vi "Configure List Parameters.vi"(0 "VISA resource name":refnum<visa-resource-name>, 1 "List File Number (1)":dbl=1.0 min=1.0 max=10.0 step=1.0, 2 "Address (0)":dbl min=0.0 max=31.0 step=1.0 format="%#.0p", 5 "List Power Limit (1200)":dbl=1200.0 min=1.0 max=1200.0 step=1.0, 7 "Repeat Count (1)":i32=1 min=1 max=65535 step=1, 9 "Linked Sequences (0000000000)":bool[](array[boolean])=[FALSE, FALSE, FALSE, FALSE, FALSE, FALSE, FALSE, FALSE, FALSE, FALSE], 11 "error in (no error)":errorcluster) -> (4 "VISA resource name out":refnum<visa-resource-name>, 15 "error out":errorcluster)   [LabVIEW 2020, in "BK Precision 911X Series.lvlib"]
doc: "Configures list parameters for list operation. Use this vi before running <b>Configure List Sequence Repeat.vi</b>.\n\n<b>Note: List program functionality is not available on model 9117.</b>"
uses:
  BK Precision 911X Series.lvlib
panel:
  # "Sequence #  1   2    3   4    5   6   7    8   9   0"
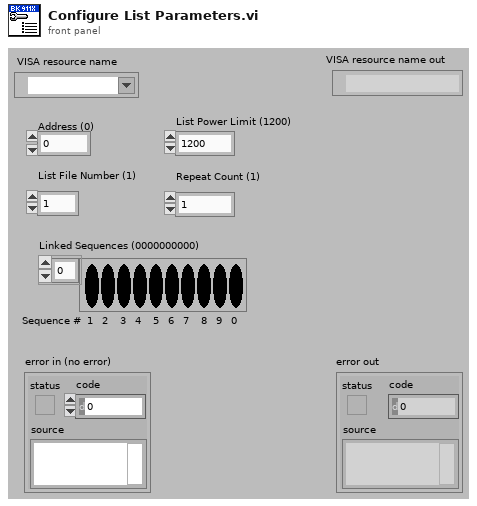
[diagram p1: front panel]
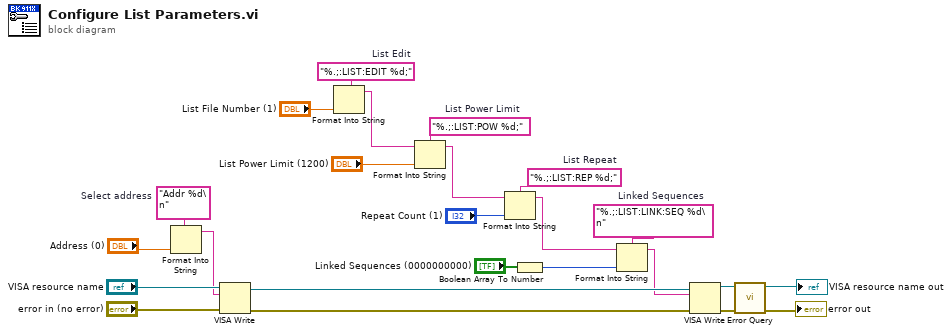
[diagram p0: block diagram]
diagram:
  w5 = "%.;:LIST:LINK:SEQ %d\n"  # Linked Sequences
  w9 = "Addr %d\n"  # Select address
  w15 = "%.;:LIST:REP %d;"  # List Repeat
  w19 = "%.;:LIST:POW %d;"  # List Power Limit
  w21 = "%.;:LIST:EDIT %d;"  # List Edit
  n1 = Format Into String(format string=w9, "Address (0)") -> (resulting string=w6:string)  [unwired: 2 in, 1 out]
  n2 = VISA Write(VISA resource name="VISA resource name", write buffer=w6, error in (no error)="error in (no error)") -> (VISA resource name out=w24:refnum<visa-resource-name>, error out=w23:errorcluster)  [unwired: 1 out]
  n3 = Format Into String(format string=w21, "List File Number (1)") -> (resulting string=w17:string)  [unwired: 2 in, 1 out]
  n4 = Format Into String(format string=w19, initial string=w17, "List Power Limit (1200)") -> (resulting string=w16:string)  [unwired: 1 in, 1 out]
  n5 = Format Into String(format string=w15, initial string=w16, "Repeat Count (1)") -> (resulting string=w4:string)  [unwired: 1 in, 1 out]
  n6 = Boolean Array To Number(Boolean array="Linked Sequences (0000000000)") -> (number=w1:u32)
  n7 = Format Into String(format string=w5, initial string=w4, w1) -> (resulting string=w3:string)  [unwired: 1 in, 1 out]
  n8 = VISA Write(VISA resource name=w24, write buffer=w3, error in (no error)=w23) -> (VISA resource name out=w13:refnum<visa-resource-name>, error out=w12:errorcluster)  [unwired: 1 out]
  n9 = call "Error Query.vi"("error in (no error)"=w12, "VISA resource name"=w13) -> ("error out"=→"error out":errorcluster, "VISA resource name out"=→"VISA resource name out":refnum<visa-resource-name>)  [unwired: 6 in, 2 out]
